vi "Sel_arr-Gauss-fit.vi"(5 "parameter bounds":T2, 6 "initial guess":T1, 7 "Cursor.Cursor Y":dbl, 8 "Cursor.Cursor X":dbl, 9 "Selection length":i32, 10 "Sub Array":dbl[][](array[numeric])) -> (0 "standard deviation":dbl, 1 "center":dbl, 2 "amplitude":dbl, 3 "Array":dbl[][](array[numeric]), 4 "Slice 2":dbl[](graph))   [LabVIEW 2017]
uses:
  <vilib>/Analysis/baseanly.llb/Mean (DBL).vi
  <vilib>/Analysis/NI_AALPro.lvlib
  <vilib>/Analysis/NI_AALBase.lvlib
panel:
  out "median":dbl format="%0.2f"
  out "mean":dbl format="%0.2f"
  out "Slice 3":dbl[](graph)
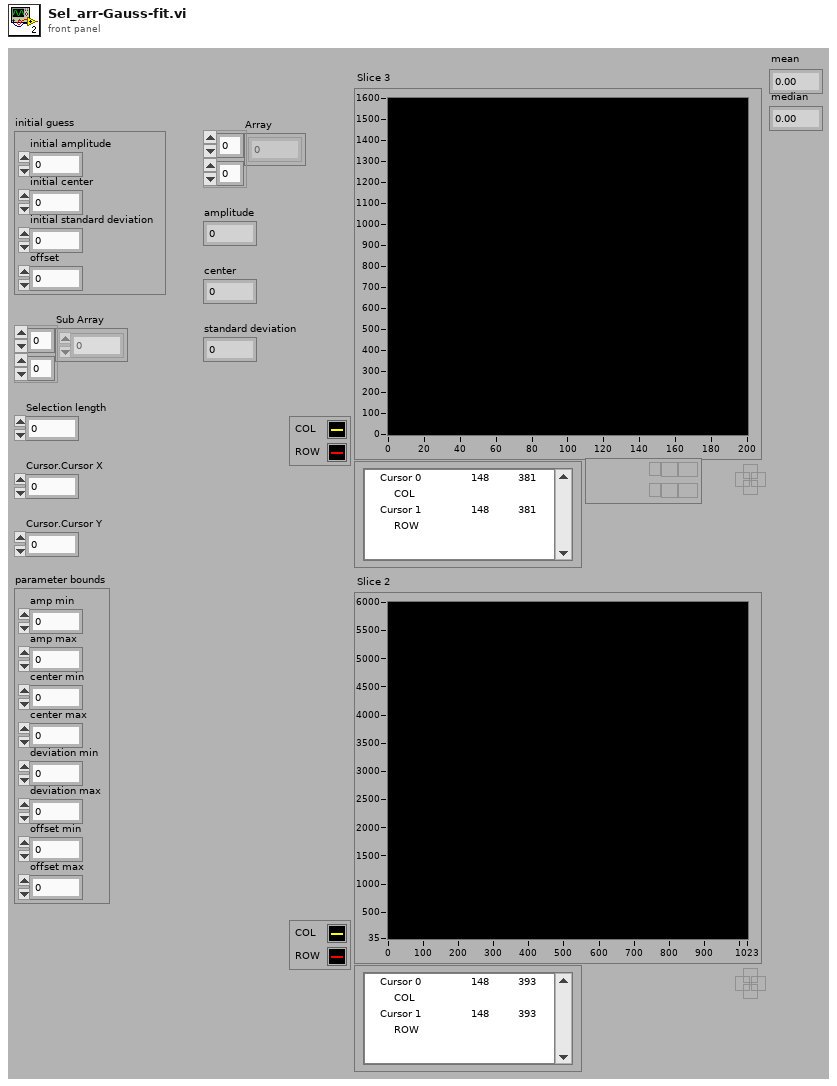
[diagram p1: front panel]
types:
  T1 = cluster{"initial amplitude":dbl, "initial center":dbl, "initial standard deviation":dbl, "offset":dbl}
  T2 = cluster{"amp min":dbl, "amp max":dbl, "center min":dbl, "center max":dbl, "deviation min":dbl, "deviation max":dbl, "offset min":dbl, "offset max":dbl}
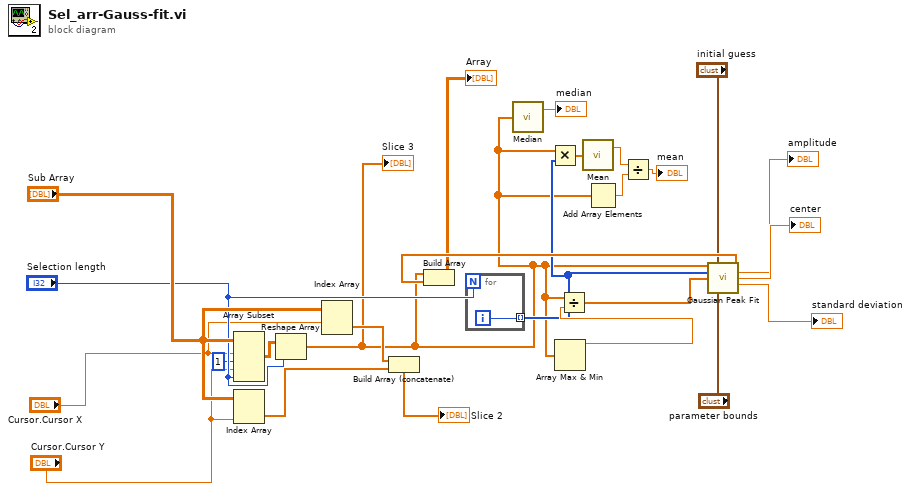
[diagram p0: block diagram]
diagram:
  n1 = Array Subset(array="Sub Array", index (row)="Cursor.Cursor X", length (row)=1 ("length"), index (col)="Cursor.Cursor Y", length (col)="Selection length") -> (w14:dbl[][])
  n2 = Index Array(array="Sub Array", index (col)="Cursor.Cursor Y") -> (element=w10:dbl[])  [unwired: 1 in]
  n3 = Reshape Array(w14, "Selection length") -> (w4:dbl[])
  "Slice 3" <- w4
  n4 = Index Array(array="Sub Array", index (row)="Cursor.Cursor X") -> (element=w8:dbl[])  [unwired: 1 in]
  n5 = Build Array (concatenate)(w8, w10) -> (→"Slice 2":dbl[])
  n6 = for {
    N: "Selection length" -> [_]
    tunnel: [w26] -> w7 mode=indexing
    i -> [w26]
  }
  n7 = call <vilib>:"Median.vi"("X"=w4) -> ("median"=→"median":dbl)  [unwired: 1 out]
  n8 = Multiply(x=w4, y=w7) -> (x*y=w6:dbl[])
  n9 = Array Max & Min(array=w4) -> (max value=w23:dbl)  [unwired: 3 out]
  n10 = Divide(x=w4, y=w23) -> (x/y=w22:dbl[])
  n11 = call-poly <vilib>:"Mean.vi"("X"=w6) -> ("mean"=w1:dbl)  [unwired: 1 out]
  n12 = Add Array Elements(numeric array=w4) -> (sum=w3:dbl)
  n13 = Divide(x=w1, y=w3) -> (x/y=→"mean":dbl)
  n14 = call <vilib>:"Gaussian Peak Fit.vi"("Y"=w4, "initial guess"="initial guess", "X"=w7, "Weight"=w22, "parameter bounds"="parameter bounds") -> ("Best Gaussian Fit"=w21:dbl[], "amplitude"=→"amplitude":dbl, "center"=→"center":dbl, "standard deviation"=→"standard deviation":dbl)  [unwired: 4 in, 3 out]
  n15 = Build Array(w4, w21) -> (→"Array":dbl[][])
